vi "parse binary file header.vi"(8 "error in":errorcluster, 11 "Byte Stream File in":refnum<file>) -> (0 "error out":errorcluster, 1 "data":T1[](array[typedef]), 2 "dictionary":T3, 3 "Byte Stream File out":refnum<file>, 4 "remaining string":string, 5 "version":string)   [LabVIEW 2013, in "Binary datalogger runtime.lvclass"]
uses:
  Binary datalogger runtime.lvclass
  <vilib>/NI/Tag Bus/dictionary/full data dictionary.ctl
  data cache.ctl
  <vilib>/NI/Tag Bus/table/data table.ctl
  <vilib>/NI/Tag Bus/table/data table.lvlib
  <vilib>/NI/Tag Bus/dictionary/data dictionary.lvclass
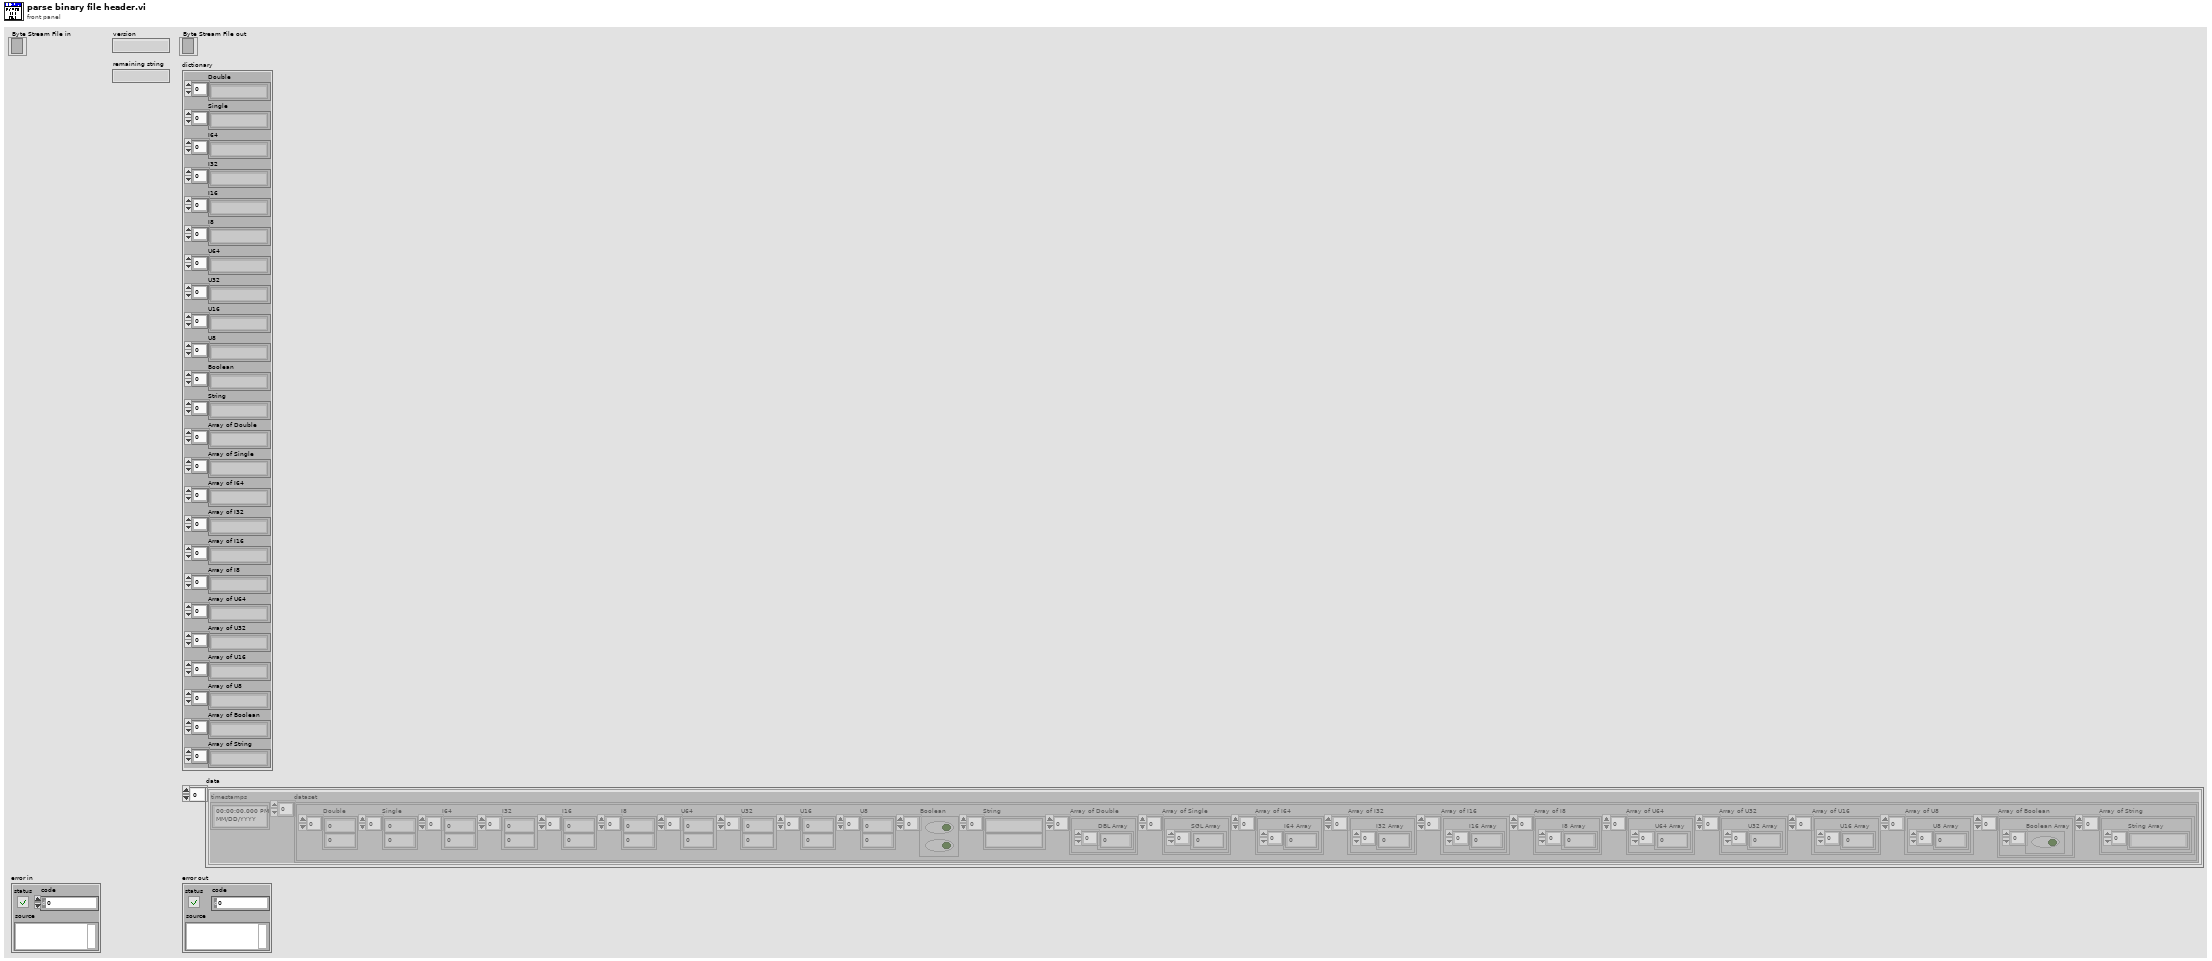
[diagram p1: front panel]
types:
  T1 = typedef "Binary datalogger runtime.lvclass/data cache.ctl" = cluster{"timestamps":timestamp[], "dataset":T2[]}
  T2 = typedef "tag bus.lvlib/data table.lvlib/data table.ctl" = cluster{"Double":dbl[], "Single":sgl[], "I64":i64[], "I32":i32[], "I16":i16[], "I8":i8[], "U64":u64[], "U32":u32[], "U16":u16[], "U8":u8[], "Boolean":bool[], "String":string[], "Array of Double":cluster{"DBL Array":dbl[]}[], "Array of Single":cluster{"SGL Array":sgl[]}[], "Array of I64":cluster{"I64 Array":i64[]}[], "Array of I32":cluster{"I32 Array":i32[]}[], "Array of I16":cluster{"I16 Array":i16[]}[], "Array of I8":cluster{"I8 Array":i8[]}[], "Array of U64":cluster{"U64 Array":u64[]}[], "Array of U32":cluster{"U32 Array":u32[]}[], "Array of U16":cluster{"U16 Array":u16[]}[], "Array of U8":cluster{"U8 Array":u8[]}[], "Array of Boolean":cluster{"Boolean Array":bool[]}[], "Array of String":cluster{"String Array":string[]}[]}
  T3 = typedef "tag bus.lvlib/data dictionary.lvclass/full data dictionary.ctl" = cluster{"Double":string[], "Single":string[], "I64":string[], "I32":string[], "I16":string[], "I8":string[], "U64":string[], "U32":string[], "U16":string[], "U8":string[], "Boolean":string[], "String":string[], "Array of Double":string[], "Array of Single":string[], "Array of I64":string[], "Array of I32":string[], "Array of I16":string[], "Array of I8":string[], "Array of U64":string[], "Array of U32":string[], "Array of U16":string[], "Array of U8":string[], "Array of Boolean":string[], "Array of String":string[]}
  T4 = cluster{"Double":string[], "Single":string[], "I64":string[], "I32":string[], "I16":string[], "I8":string[], "U64":string[], "U32":string[], "U16":string[], "U8":string[], "Boolean":string[], "String":string[], "Array of Double":string[], "Array of Single":string[], "Array of I64":string[], "Array of I32":string[], "Array of I16":string[], "Array of I8":string[], "Array of U64":string[], "Array of U32":string[], "Array of U16":string[], "Array of U8":string[], "Array of Boolean":string[], "Array of String":string[]}
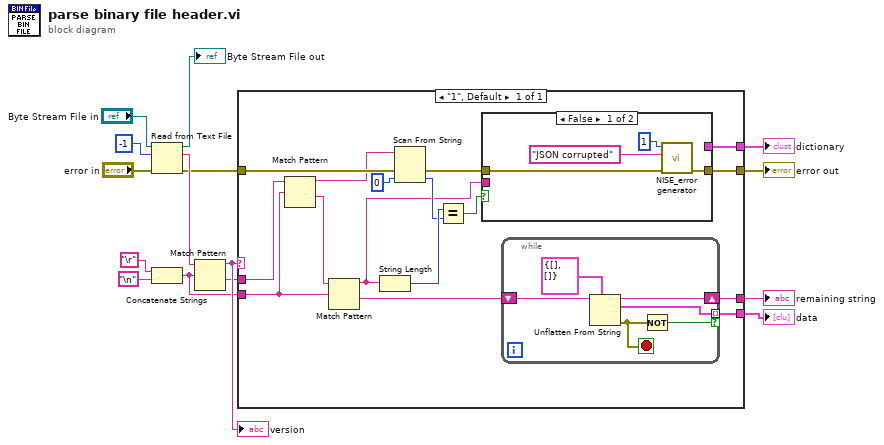
[diagram p0: block diagram]
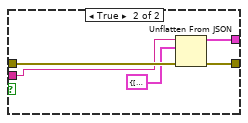
[diagram p2: hidden frame]
diagram:
  n1 = Read from Text File(file (use dialog)="Byte Stream File in", count=-1, error in="error in") -> (refnum out=→"Byte Stream File out":refnum<file>, text=w11:string, error out=w6:errorcluster)  [unwired: 1 in, 1 out]
  n2 = Concatenate Strings("\r", "\n") -> (w4:string)
  n3 = Match Pattern(string=w11, regular expression=w4) -> (before substring=w8:string, after substring=w5:string)  [unwired: 1 in, 2 out]
  "version" <- w8
  n4 = case shown="\"1\", Default" w8 {
    tunnel: [w21] -> w7
    tunnel: w6 -> [w31]
    tunnel: w5 -> [w30]
    tunnel: w4 -> [w26]
    tunnel: [w20] -> w3
    tunnel: [w17] -> w2
    tunnel: [w16] -> w1
    frame "1", Default {
      n5 = Match Pattern(string=w30, regular expression=w26) -> (before substring=w28:string, after substring=w27:string)  [unwired: 1 in, 2 out]
      n6 = Match Pattern(string=w27, regular expression=w26) -> (before substring=w19:string, after substring=w18:string)  [unwired: 1 in, 2 out]
      n7 = String Length(string=w19) -> (length=w25:i32)
      n8 = Scan From String(input string=w28, error in=w31, default 1=0 ("length")) -> (error out=w22:errorcluster, output 1=w24:i32)  [unwired: 2 in, 2 out]
      n9 = Equal?(x=w25, y=w24) -> (x = y?=w23:bool)
      n10 = case shown="False" w23 {
        tunnel: w22 -> [w41 w46]
        tunnel: [w40 w45] -> w21
        tunnel: [_ w43] -> w20
        tunnel: w19 -> [_ w42]
        frame False {
          n11 = call <vilib>:"NISE_error generator.vi"("error in"=w41, "append error message"="JSON corrupted", "error code (0)"=1) -> ("error out"=w40:errorcluster)  [unwired: 6 in]
        }
        frame True {
          n12 = Unflatten From JSON(JSON string=w42, type and defaults=T4 {"Double"=[], "Single"=[], "I64"=[], "I32"=[], "I16"=[], "I8"=[], "U64"=[], "U32"=[], "U16"=[], "U8"=[], "Boolean"=[], "String"=[], "Array of Double"=[], "Array of Single"=[], "Array of I64"=[], "Array of I32"=[], "Array of I16"=[], "Array of I8"=[], "Array of U64"=[], "Array of U32"=[], "Array of U16"=[], "Array of U8"=[], "Array of Boolean"=[], "Array of String"=[]} ("dictionary"), error in (no error)=w46) -> (value=w43:T4, error out=w45:errorcluster)  [unwired: 4 in]
        }
      }
      n13 = while {
        shift-right: [w35] -> w16
        shift-left: w18 -> [w36]
        tunnel: [w34] -> w17 mode=indexing if=w32
        stop <- w33 stop-if-true
        n14 = Unflatten From String(type=T1 {"timestamps"=[], "dataset"=[]} ("dataset"), binary string=w36) -> (rest of the binary string=w35:string, value=w34:T1, error out=w33:errorcluster)  [unwired: 3 in]
        n15 = Not(x=w33) -> (.not. x?=w32:bool)
      }
    }
  }
  "dictionary" <- w3
  "error out" <- w7
  "data" <- w2
  "remaining string" <- w1
